vi "FileIO-Read Parameters.vi"(0 "Settings file":path, 1 "Type of Parameters":variant, 7 "Default Folder":path, 9 "Prompt?":bool, 11 "error in (no error)":errorcluster) -> (4 "Path out":path, 6 "Anything":variant, 8 "Version":i32, 10 "Read?":bool, 15 "error out":errorcluster)   [LabVIEW 2020]
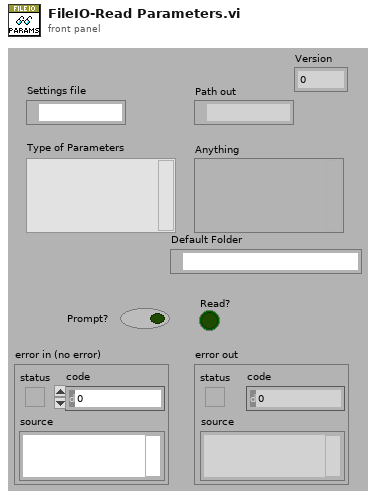
[diagram p1: front panel]
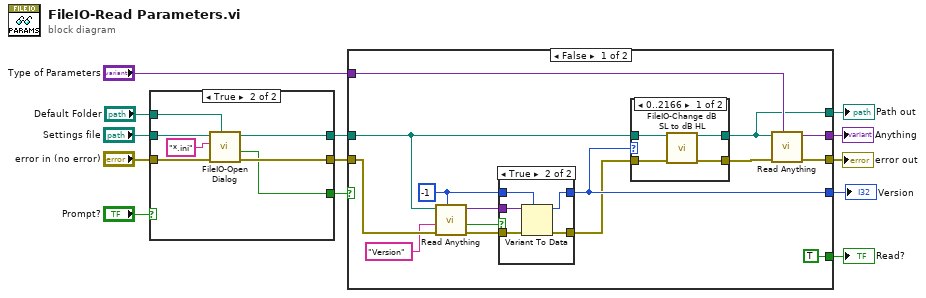
[diagram p0: block diagram]
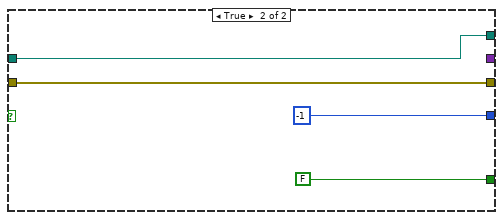
[diagram p4: hidden frame]
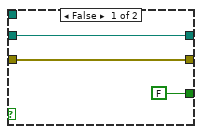
[diagram p5: hidden frame]
diagram:
  n1 = case shown="True" "Prompt?" {
    tunnel: "Settings file" -> [w16 w23]
    tunnel: "error in (no error)" -> [w15 w21]
    tunnel: [w15 w20] -> w9
    tunnel: [w16 w19] -> w8
    tunnel: [FALSE ("cancelled") w18] -> w10
    tunnel: "Default Folder" -> [_ w17]
    frame False {
    }
    frame True {
      n2 = call "FileIO-Open Dialog.vi"("Default Folder"=w17, "error in"=w21, "pattern (all files)"="*.ini", "Start path"=w23) -> ("error out"=w20:errorcluster, "cancelled"=w18:bool, "selected path"=w19:path)  [unwired: 5 in]
    }
  }
  n3 = case shown="False" w10 {
    tunnel: w9 -> [w34 w55]
    tunnel: w8 -> [w26 w53]
    tunnel: [w38 _] -> w5
    tunnel: [w37 w55] -> w7
    tunnel: [TRUE FALSE] -> w6
    tunnel: [w27 w53] -> w4
    tunnel: "Type of Parameters" -> [w35 _]
    tunnel: [w28 -1] -> w1
    frame False {
      w30 = -1
      n4 = call "Read Anything.vi"("Type of Anything"=w30, "Error In"=w34, "Section Name (Name of \"Type of Anything\")"="Version" ("Section Name (Name of \"Type of Anything\")"), "Path (dialog)"=w26) -> ("Error Out"=w29:errorcluster, "Found?"=w32:bool, "Anything"=w31:variant)  [unwired: 5 in]
      n5 = case shown="True" w32 {
        tunnel: w31 -> [_ w51]
        tunnel: w30 -> [w46 w50]
        tunnel: [w46 w49] -> w28
        tunnel: w29 -> [w45 w48]
        tunnel: [w45 w47] -> w25
        frame False {
        }
        frame True {
          n6 = Variant To Data(error in=w48, type=w50, Variant=w51) -> (data=w49:i32, error out=w47:errorcluster)
        }
      }
      n7 = case shown="0..2166" w28 {
        tunnel: [w42 w44] -> w27
        tunnel: w26 -> [w41 w44]
        tunnel: w25 -> [w40 w43]
        tunnel: [w39 w43] -> w24
        frame 0..2166 {
          n8 = call "FileIO-Change dB SL to dB HL.vi"("selected path in"=w41, "error in (no error)"=w40) -> ("selected path out"=w42:path, "error out"=w39:errorcluster)  [unwired: 12 in]
        }
        frame 2167, Default {
        }
      }
      n9 = call "Read Anything.vi"("Type of Anything"=w35, "Error In"=w24, "Path (dialog)"=w27) -> ("Error Out"=w37:errorcluster, "Anything"=w38:variant)  [unwired: 6 in, 1 out]
    }
    frame True {
    }
  }
  "error out" <- w7
  "Read?" <- w6
  "Path out" <- w4
  "Anything" <- w5
  "Version" <- w1
